vi "Read Port Configuration.vi"(8 "error in (no error)":errorcluster, 11 "CAN_Logic in":refnum<class "CAN_Logic.lvclass">) -> (0 "error out":errorcluster, 2 "CAN Port Config":T1={"Mode"=enum."CAN FD", "Baud Rate"=500000, "Temination On"=TRUE, "Subordinate"=FALSE, "Echo TX"=FALSE, "FD Config"={"FD Baud Rate"=2000000, "ISO Mode"=TRUE, "BRS Enabled"=TRUE}} {"FD Config"."FD Baud Rate" format="%.0p"; "Baud Rate" format="%.0p"}, 3 "CAN_Logic out":refnum<class "CAN_Logic.lvclass">)   [LabVIEW 2021, in "CAN_Logic.lvclass"]
uses:
  CAN_Logic.lvclass
  CAN_Logic.lvclass/CAN_Logic.ctl
  typedef/CAN Mode.ctl
  typedef/FD Config.ctl
  typedef/CAN Port Configuration.ctl
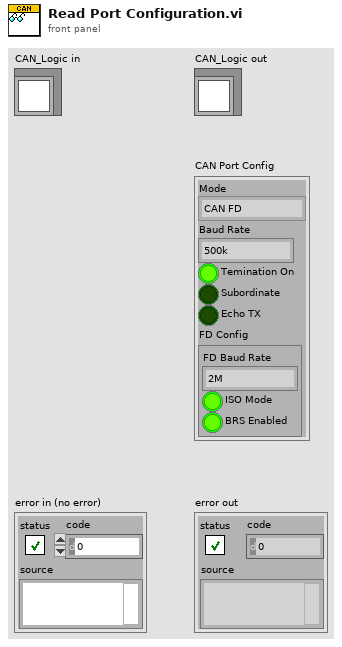
[diagram p1: front panel]
types:
  T1 = typedef "CAN_Logic.lvclass/CAN Port Configuration.ctl" = cluster{"Mode":T2, "Baud Rate":u64, "Temination On":bool, "Subordinate":bool, "Echo TX":bool, "FD Config":T3}
  T2 = typedef "CAN_Logic.lvclass/CAN Mode.ctl" = enum16{"CAN 2.0", "CAN FD"}
  T3 = typedef "CAN_Logic.lvclass/FD Config.ctl" = cluster{"FD Baud Rate":u64, "ISO Mode":bool, "BRS Enabled":bool}
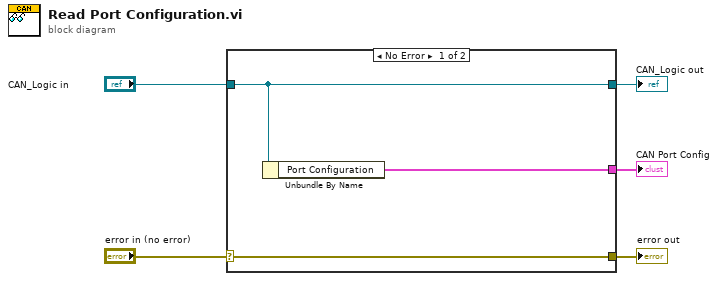
[diagram p0: block diagram]
diagram:
  n1 = case shown="No Error" "error in (no error)" {
    selector: "error in (no error)" -> [w8 w9]
    tunnel: [w8 w9] -> w4
    tunnel: [w7 w10] -> w2
    tunnel: "CAN_Logic in" -> [w7 w10]
    tunnel: [w6 _] -> w1
    frame No Error {
      n2 = Unbundle By Name(w7) -> ("Port Configuration"=w6:T1)
    }
    frame Error {
    }
  }
  "error out" <- w4
  "CAN_Logic out" <- w2
  "CAN Port Config" <- w1
